vi "GetSimpleArray.vi"(8 "error in":errorcluster, 9 "ArraySize":i32, 10 "Tag":string, 11 "node in":refnum<k20>) -> (0 "error out":errorcluster, 2 "TextArray":string[](array[string]), 3 "node out":refnum<k20>)   [LabVIEW 2010, in "Pansino_XML_Read.lvlib"]
uses:
  <vilib>/xml/Close Reference(Node).vi
  Pansino_XML_Read.lvlib
  <vilib>/xml/NI_XML.lvlib
  C:/Program Files (x86)/National Instruments/LabVIEW 2010/resource/objmgr/DOMUserDefRef.rc
panel:
  out "Has Child Nodes":bool
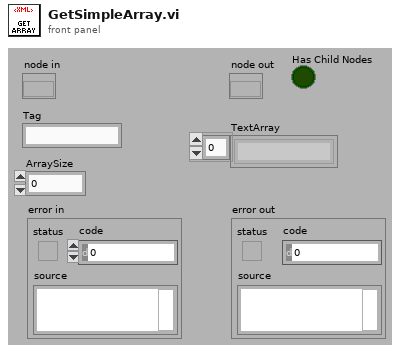
[diagram p1: front panel]
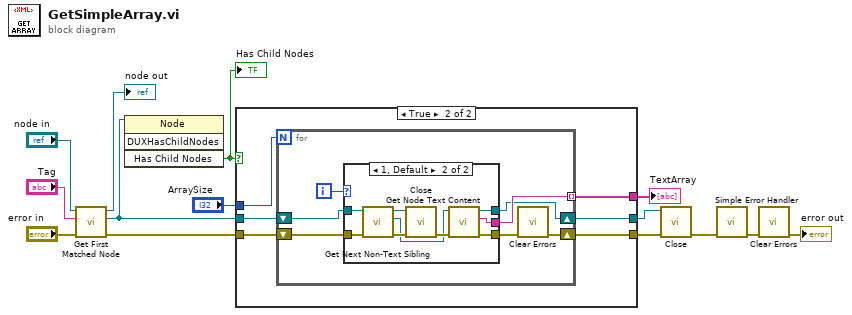
[diagram p0: block diagram]
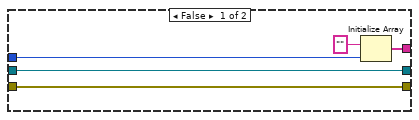
[diagram p2: hidden frame]
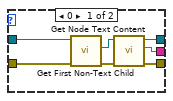
[diagram p3: hidden frame]
diagram:
  n1 = call <vilib>:"Get First Matched Node.vi"("error in (no error)"="error in", "XPath expression"="Tag", "node in"="node in") -> ("error out"=w12:errorcluster, "node result"=w6:refnum<k20>, "node out"=→"node out":refnum<k20>)  [unwired: 6 in]
  n2 = invoke class="Node" method="DUXHasChildNodes"(reference=w6) -> ("Has Child Nodes"=w5:bool)  [unwired: 3 in, 3 out]
  "Has Child Nodes" <- w5
  n3 = case shown="True" w5 {
    tunnel: [w18 w25] -> w4
    tunnel: [w19 w24] -> w3
    tunnel: "ArraySize" -> [w17 w23]
    tunnel: w6 -> [w18 w22]
    tunnel: w12 -> [w19 w21]
    tunnel: [w16 w20] -> w7
    frame False {
      n4 = Initialize Array("" ("node text"), w17) -> (w16:string[])
    }
    frame True {
      n5 = for {
        N: w23 -> [_]
        tunnel: [w32] -> w20 mode=indexing
        shift-right: [w26] -> w24
        shift-left: w21 -> [w31]
        shift-right: [w29] -> w25
        shift-left: w22 -> [w30]
        i -> [w28]
        n6 = case shown="1, Default" w28 {
          tunnel: [w38 w44] -> w27
          tunnel: [w37 w43] -> w32
          tunnel: w31 -> [w34 w42]
          tunnel: w30 -> [w36 w41]
          tunnel: [w39 w40] -> w29
          frame 0 {
            n7 = call <vilib>:"Get First Non-Text Child.vi"("error in (no error)"=w34, "node in"=w36) -> ("error out"=w33:errorcluster, "child node"=w35:refnum<k20>)  [unwired: 6 in, 2 out]
            n8 = call <vilib>:"Get Node Text Content.vi"("error in (no error)"=w33, "node in"=w35) -> ("error out"=w38:errorcluster, "node text"=w37:string, "node out"=w39:refnum<k20>)  [unwired: 7 out]
          }
          frame 1, Default {
            n9 = call <vilib>:"Get Next Non-Text Sibling.vi"("error in (no error)"=w42, "node in"=w41) -> ("error out"=w47:errorcluster, "sibling node"=w45:refnum<k20>, "node out"=w46:refnum<k20>)  [unwired: 7 out]
            n10 = call-poly <vilib>:"Close.vi"("error in (no error)"=w47, "node"=w46) -> ("error out"=w48:errorcluster)  [unwired: 7 out]
            n11 = call <vilib>:"Get Node Text Content.vi"("error in (no error)"=w48, "node in"=w45) -> ("error out"=w44:errorcluster, "node text"=w43:string, "node out"=w40:refnum<k20>)  [unwired: 7 out]
          }
        }
        n12 = call <vilib>:"Clear Errors.vi"("error in (no error)"=w27) -> ("error out"=w26:errorcluster)  [unwired: 6 in]
      }
    }
  }
  "TextArray" <- w7
  n13 = call-poly <vilib>:"Close.vi"("error in (no error)"=w3, "node"=w4) -> ("error out"=w14:errorcluster)  [unwired: 7 out]
  n14 = call <vilib>:"Simple Error Handler.vi"("error in (no error)"=w14) -> ("error out"=w2:errorcluster)  [unwired: 4 in, 4 out]
  n15 = call <vilib>:"Clear Errors.vi"("error in (no error)"=w2) -> ("error out"=→"error out":errorcluster)  [unwired: 6 in]
